vi "Status Decoder.vi"() -> ()   [LabVIEW 2020]
panel:
  out "Table Control":string[][](table)
  out "Binary":u32 format="%017b"
  in  "State":u32
  # "State Decoder v1.2.14"
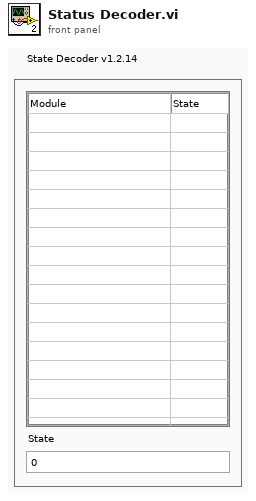
[diagram p1: front panel]
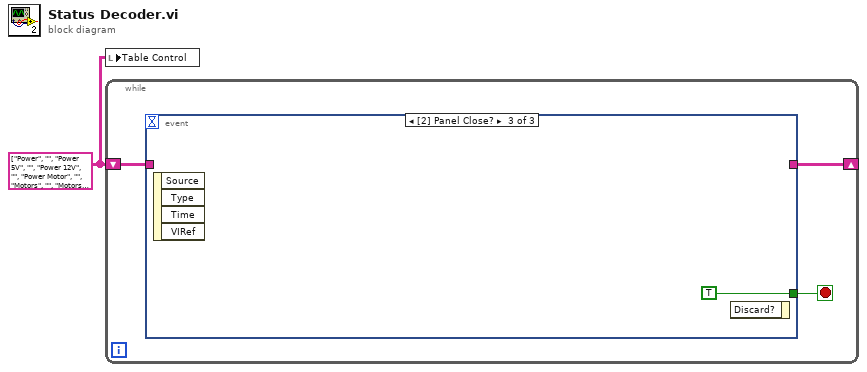
[diagram p0: block diagram]
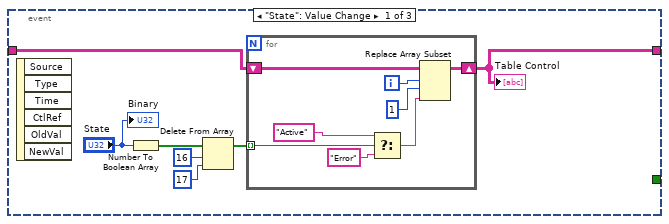
[diagram p2: hidden frame]
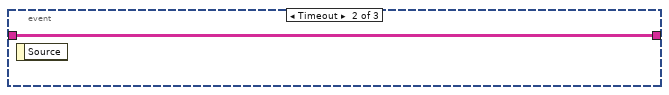
[diagram p3: hidden frame]
diagram:
  w1 = string[][] [["Power", ""], ["Power 5V", ""], ["Power 12V", ""], ["Power Motor", ""], ["Motors", ""], ["Motors State", ""], ["CANbus", ""], ["RF", ""], ["Iridium", ""], ["GNSS", ""], ["Accelerometer", ""], ["SD Card", ""], ["Blackbox", ""], ["Debug Com", ""], ["Backup CPU", ""], ["Emergency Stop", ""], ["Reserved", "Active"]] ("Table Control")
  n1 = local write "Table Control"(w1) -> ()
  n2 = while {
    shift-right: [w3] -> _
    shift-left: w1 -> [w4]
    stop <- w2 stop-if-true
    n3 = event shown="[2] Panel Close?" {
      selector: _ -> [_ _ _]
      dyn-events: _ -> [_ _ _]
      timeout: _ -> [_ _ _]
      tunnel: w4 -> [w9 w20 _]
      tunnel: [w8 w20 _] -> w3
      tunnel: [_ _ TRUE ("Discard?")] -> w2
      event "State": Value Change {
        n4 = event-data() -> ()  [unwired: 1 in, 6 out]
        n5 = Number To Boolean Array(number="State") -> (Boolean array=w10:bool[])
        n6 = Delete From Array(array=w10, length=16, index=17) -> (array with subset deleted=w5:bool[])  [unwired: 1 out]
        n7 = for {
          tunnel: w5 -> [w19] mode=indexing
          shift-right: [w16] -> w8
          shift-left: w9 -> [w15]
          i -> [w14]
          n8 = Select(t="Active", s=w19, f="Error") -> (s? t:f=w12:string)
          n9 = Replace Array Subset(array=w15, new element=w12, index (row)=w14, index (col)=1 ("index")) -> (w16:string[][])
        }
        "Table Control" <- w8
        "Binary" <- "State"
      }
      event Timeout {
        n10 = event-data() -> ()  [unwired: 1 in, 1 out]
      }
      event Panel Close? {
        n11 = event-data() -> ()  [unwired: 1 in, 4 out]
        n12 = event-data() -> ()  [unwired: 2 in, 1 out]
      }
    }
  }
